vi "#168_MAV_MSG_WIND_DECODE.vi"(11 "mavlink_payload":u8[](array[numeric])) -> (3 "WIND":T1)   [LabVIEW 2023]
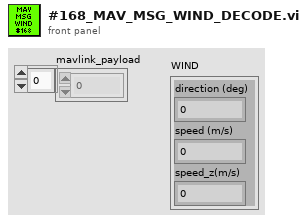
[diagram p1: front panel]
types:
  T1 = cluster{"direction (deg)":sgl, "speed (m/s)":sgl, "speed_z(m/s)":sgl}
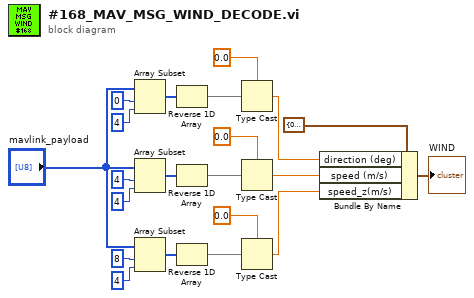
[diagram p0: block diagram]
diagram:
  n1 = Array Subset(array="mavlink_payload", index=0 ("Index"), length=4) -> (w18:u8[])
  n2 = Array Subset(array="mavlink_payload", index=4 ("Index"), length=4) -> (w12:u8[])
  n3 = Array Subset(array="mavlink_payload", index=8 ("Index"), length=4) -> (w7:u8[])
  n4 = Reverse 1D Array(array=w18) -> (reversed array=w17:u8[])
  n5 = Reverse 1D Array(array=w12) -> (reversed array=w11:u8[])
  n6 = Reverse 1D Array(array=w7) -> (reversed array=w6:u8[])
  n7 = Type Cast(type=sgl 0.0 ("Index"), x=w17) -> (*(type *) &x=w14:sgl)
  n8 = Type Cast(type=sgl 0.0 ("Index"), x=w11) -> (*(type *) &x=w1:sgl)
  n9 = Type Cast(type=sgl 0.0 ("Index"), x=w6) -> (*(type *) &x=w2:sgl)
  n10 = Bundle By Name(cluster=T1 {"direction (deg)"=0.0, "speed (m/s)"=0.0, "speed_z(m/s)"=0.0} ("WIND"), "direction (deg)"=w14, "speed (m/s)"=w1, "speed_z(m/s)"=w2) -> (→"WIND":T1)
